vi "Set Group LogType Filter.vi"(8 "error in (no error)":errorcluster, 10 "Group:CSM":string[](array[string]), 11 "GlobalLogFilter in":refnum<class "GlobalLogFilter.lvclass">) -> (0 "error out":errorcluster, 3 "GlobalLogFilter out":refnum<class "GlobalLogFilter.lvclass">)   [LabVIEW 2017, in "GlobalLogFilter.lvclass"]
uses:
  GlobalLogFilter.lvclass
  GlobalLogFilter.lvclass/GlobalLogFilter.ctl
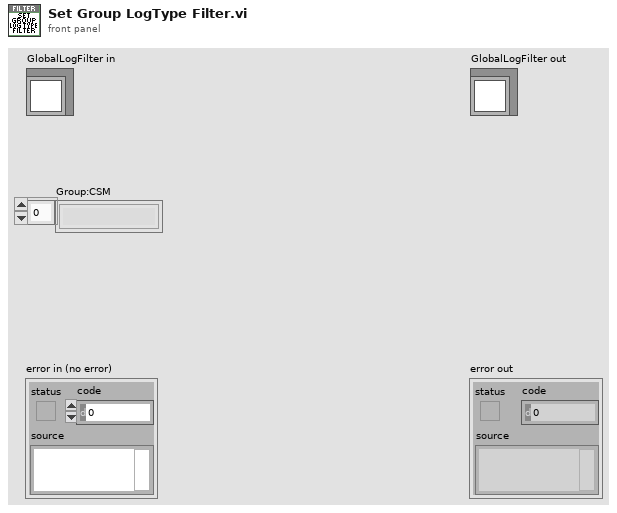
[diagram p1: front panel]
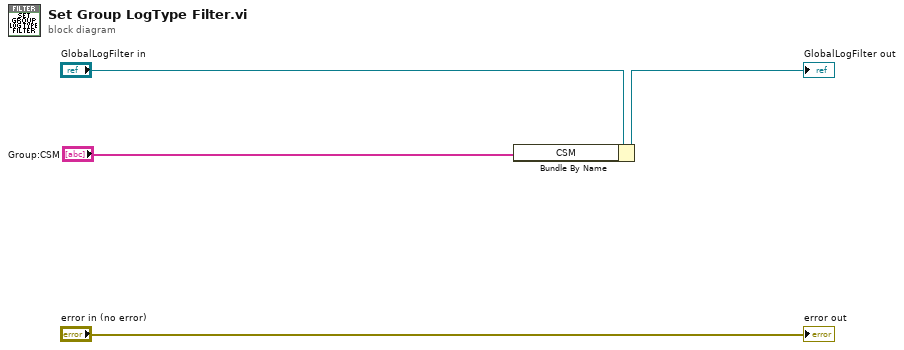
[diagram p0: block diagram]
diagram:
  n1 = Bundle By Name(cluster="GlobalLogFilter in", "CSM"="Group:CSM") -> (→"GlobalLogFilter out":refnum<class "GlobalLogFilter.lvclass">)
  "error out" <- "error in (no error)"
